vi "Customer-Panel.vi"() -> ()   [LabVIEW 2021]
uses:
  Global-Var-Simulator.vi
panel:
  out "dry_n_shine_ind":bool
  out "rinse_ind":bool
  out "soap_wash_ind":bool
  out "init_wash_ind":bool
  out "none_wash_ind":bool
  out "is_alarm_state_L":bool
  out "is_running_L":bool
  in  "none_wash_opt_btn":bool
  in  "dry_and_shine_opt_btn":bool
  in  "rinse_opt_btn":bool
  in  "soap_wash_opt_btn":bool
  in  "initial_wash_opt_btn":bool
  in  "stop_wash_btn":bool
  in  "start_wash_btn":bool
  out "seconds_ind":dbl
  out "minutes_ind":dbl
  in  "change_collect_btn":bool
  out "is_change_ready_to_collect":bool
  out "change_out_ind":dbl format="%#.2g"
  in  "home_btn":bool
  in  "cash_cancel_btn":bool
  in  "cash_accept_btn":bool
  out "cash_in_ind":dbl format="%#.2g"
  in  "add_cash_5zl_btn":bool
  in  "add_cash_2zl_btn":bool
  in  "add_cash_1zl_btn":bool
  in  "add_chash_50gr_btn":bool
  # "Alarm"
  # "Pozostały czas"
  # "sek"
  # "min"
  # "Tryby mycia"
  # "zł"
  # "Reszta do\nodbioru"
  # "zł"
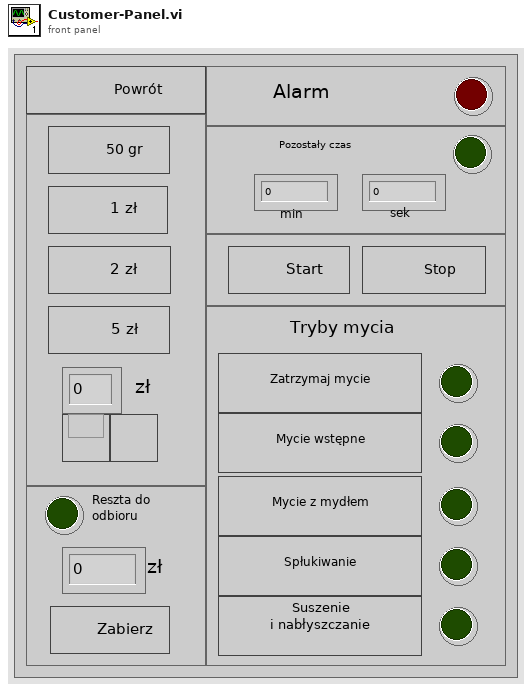
[diagram p1: front panel]
types:
  T1 = enum32{"Invalid", "Standard", "Closed", "Hidden", "Minimized", "Maximized"}
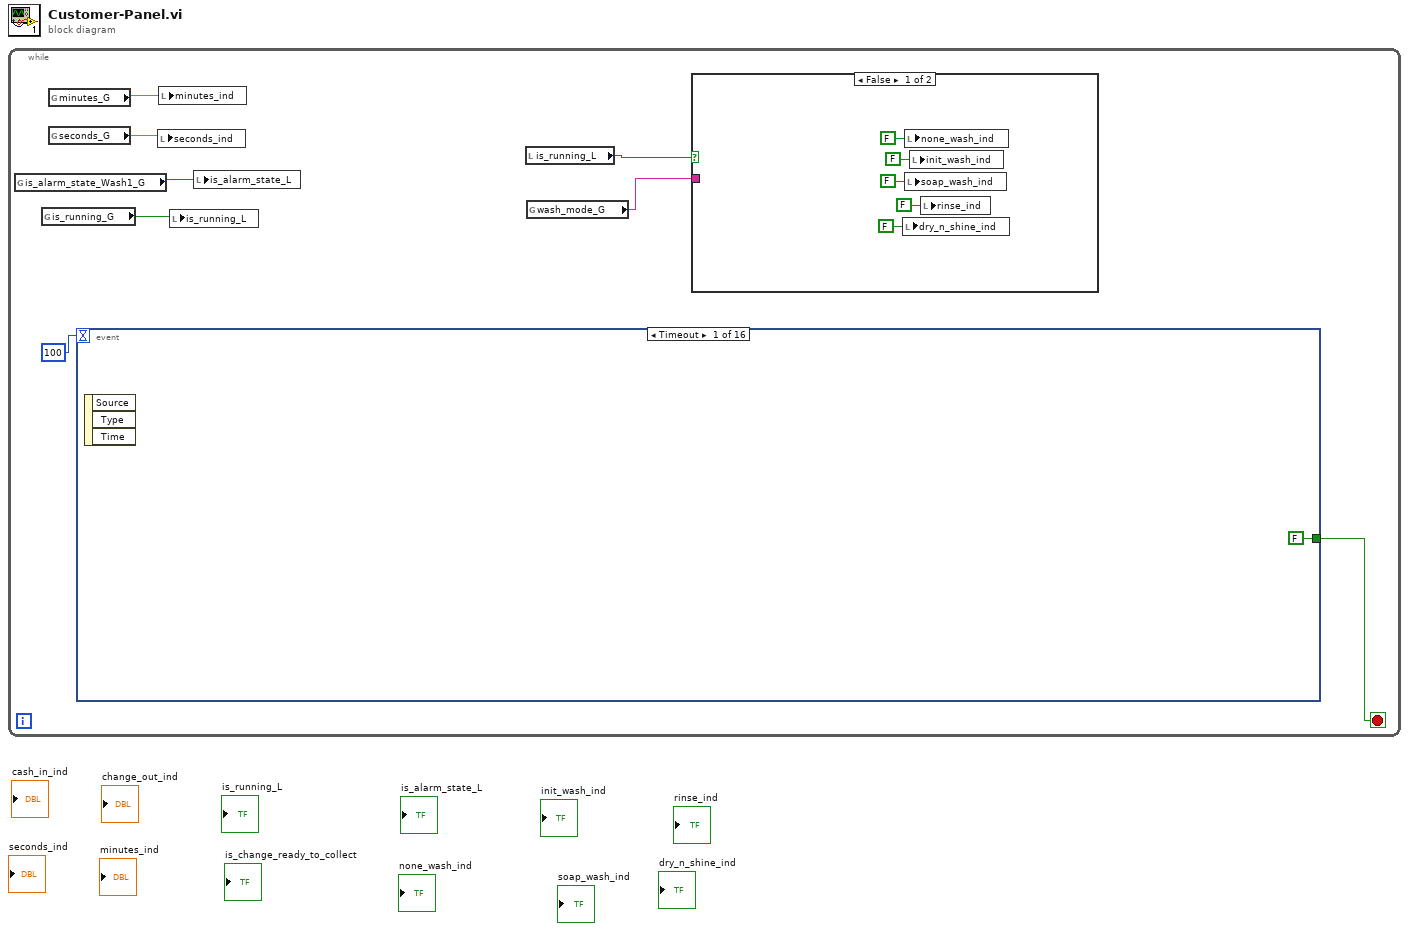
[diagram p0: block diagram]
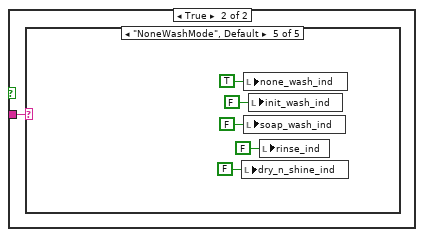
[diagram p2: hidden frame]
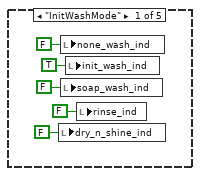
[diagram p3: hidden frame]
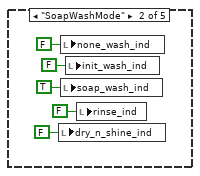
[diagram p4: hidden frame]
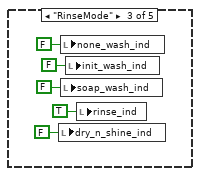
[diagram p5: hidden frame]
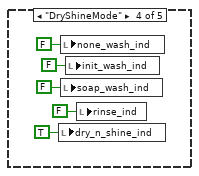
[diagram p6: hidden frame]
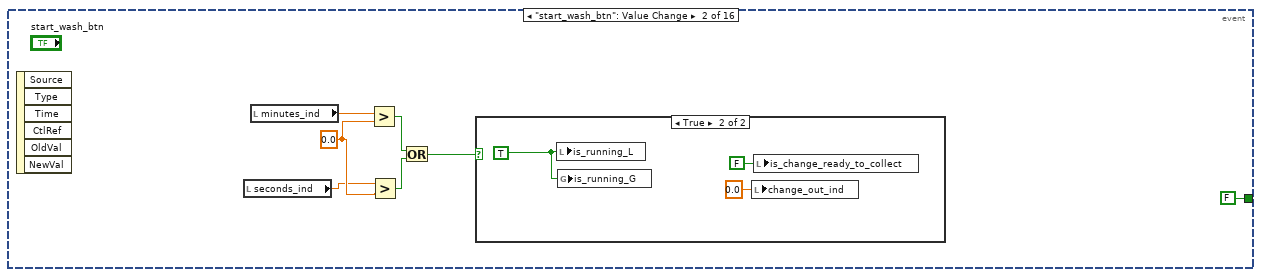
[diagram p7: hidden frame]
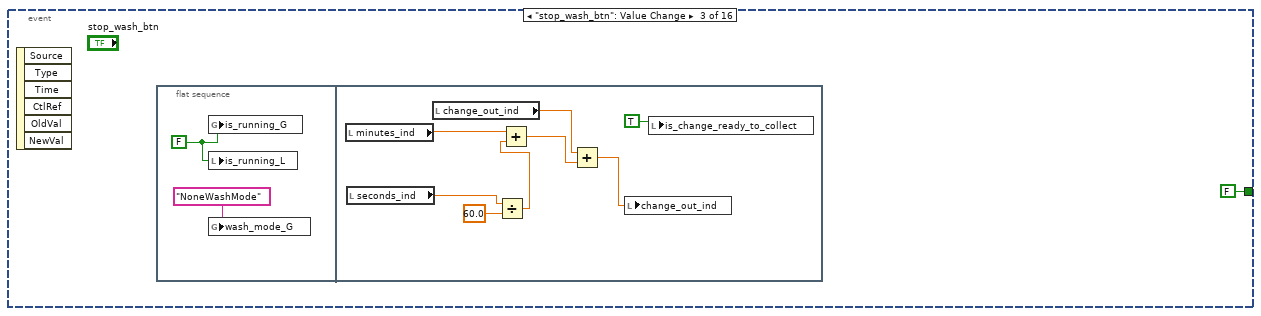
[diagram p9: hidden frame]
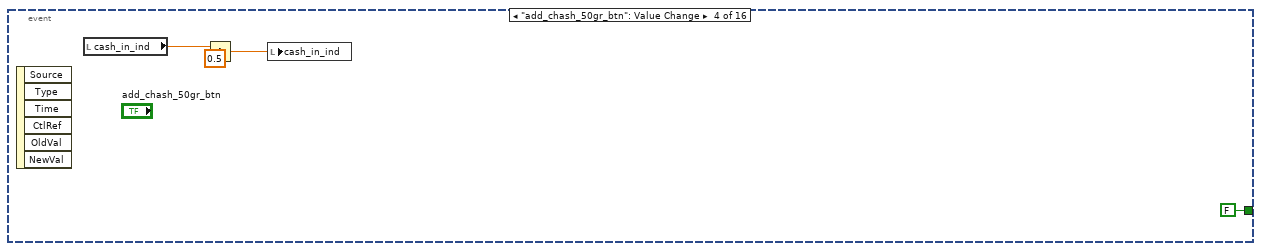
[diagram p10: hidden frame]
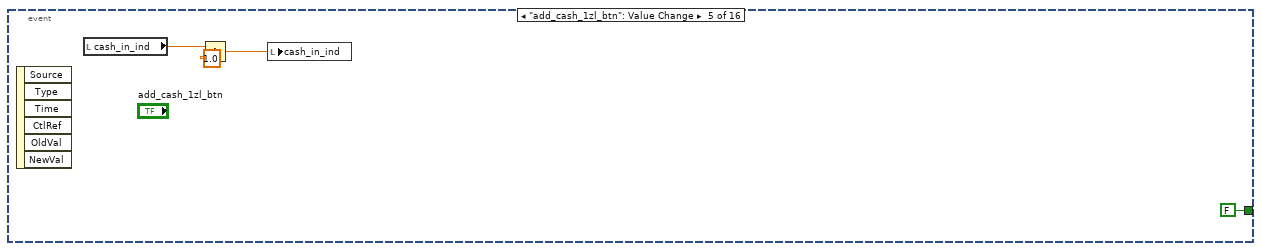
[diagram p11: hidden frame]
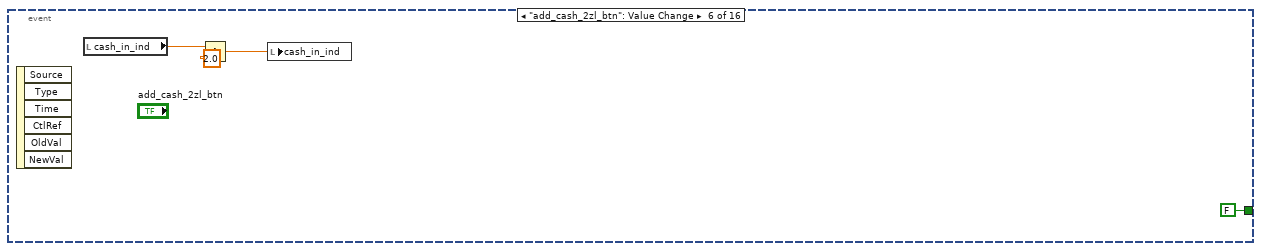
[diagram p12: hidden frame]
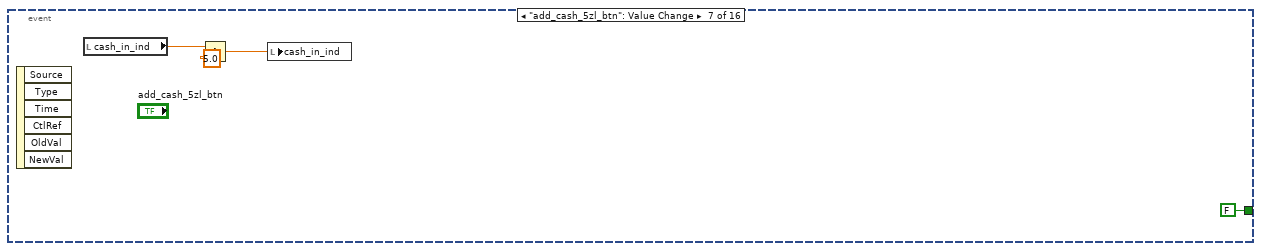
[diagram p13: hidden frame]
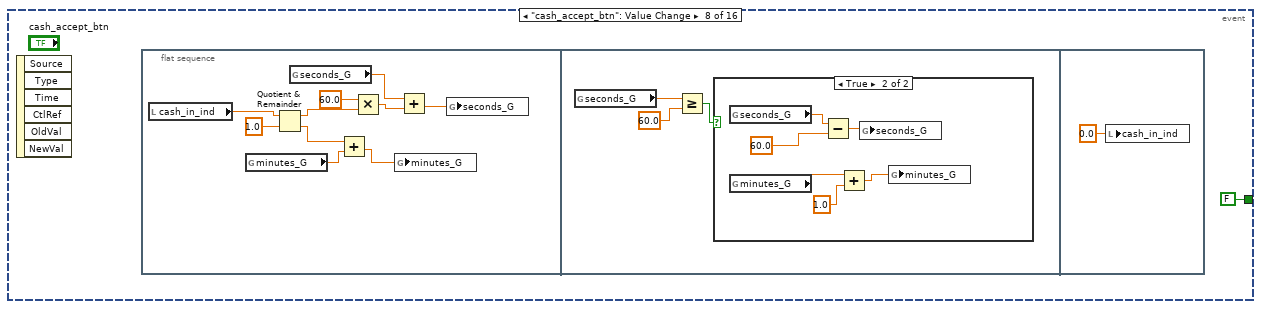
[diagram p14: hidden frame]
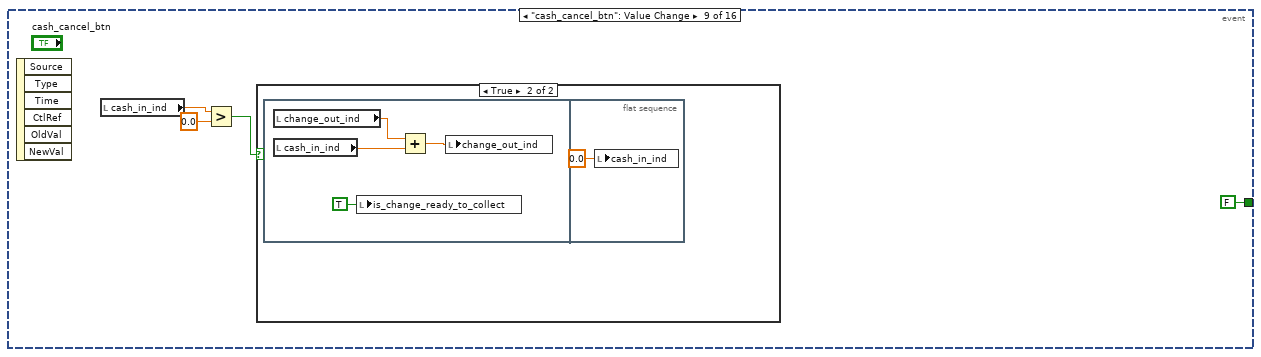
[diagram p16: hidden frame]
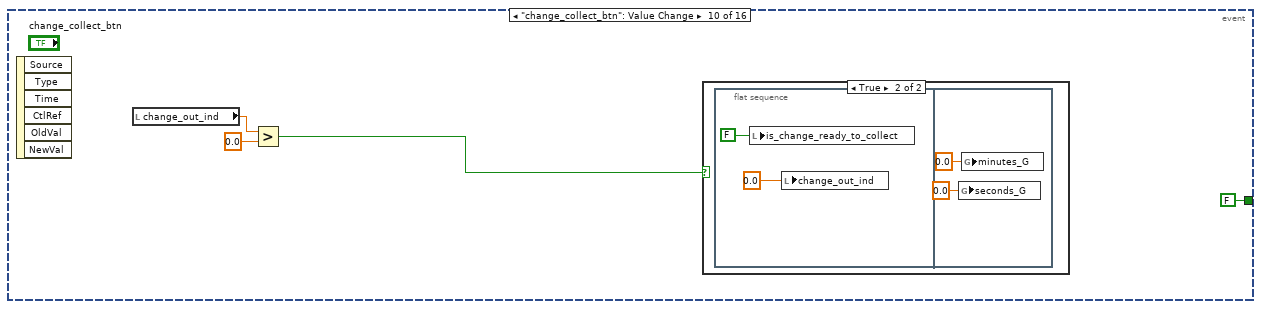
[diagram p18: hidden frame]
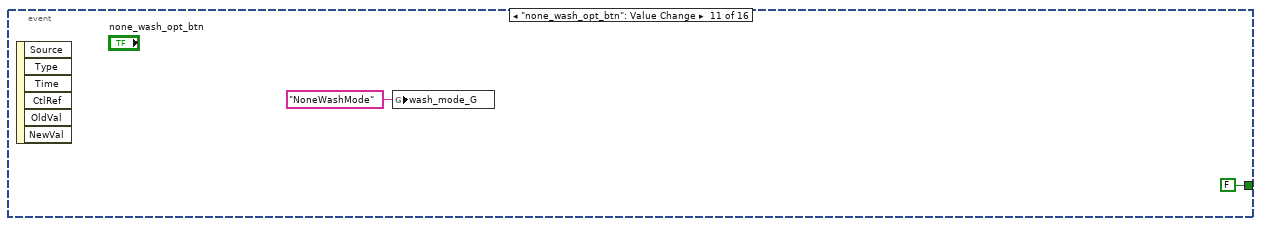
[diagram p20: hidden frame]
diagram:
  n1 = while {
    stop <- w3 stop-if-true
    n2 = global read "Global-Var-Simulator.vi" "is_alarm_state_Wash1_G"() -> (w5:bool)
    n3 = global read "Global-Var-Simulator.vi" "is_running_G"() -> (w4:bool)
    n4 = global read "Global-Var-Simulator.vi" "minutes_G"() -> (w7:dbl)
    n5 = global read "Global-Var-Simulator.vi" "seconds_G"() -> (w6:dbl)
    n6 = event shown="[0] Timeout" {
      selector: _ -> [_ _ _ _ _ _ _ _ _ _ _ _ _ _ _ _]
      dyn-events: _ -> [_ _ _ _ _ _ _ _ _ _ _ _ _ _ _ _]
      timeout: 100 -> [_ _ _ _ _ _ _ _ _ _ _ _ _ _ _ _]
      tunnel: [FALSE FALSE FALSE FALSE FALSE FALSE FALSE FALSE FALSE FALSE FALSE FALSE FALSE FALSE FALSE w126] -> w3
      event Timeout {
        n7 = event-data() -> ()  [unwired: 1 in, 3 out]
      }
      event "start_wash_btn": Value Change {
        w43 = 0.0 ("y")
        n8 = event-data() -> ()  [unwired: 1 in, 6 out]
        n9 = local read "seconds_ind"() -> (w42:dbl)
        n10 = local read "minutes_ind"() -> (w47:dbl)
        n11 = Greater?(x=w47, y=w43) -> (0:w45:bool)
        n12 = Greater?(x=w42, y=w43) -> (0:w46:bool)
        n13 = Or(x=w45, y=w46) -> (x .or. y?=w44:bool)
        n14 = case shown="True" w44 {
          frame False {
          }
          frame True {
            w50 = TRUE ("is_running_L")
            n15 = local write "is_running_L"(w50) -> ()
            n16 = global write "Global-Var-Simulator.vi" "is_running_G"(w50) -> ()
            n17 = local write "change_out_ind"(0.0 ("change_out_ind")) -> ()
            n18 = local write "is_change_ready_to_collect"(FALSE ("is_change_ready_to_collect")) -> ()
          }
        }
      }
      event "stop_wash_btn": Value Change {
        n19 = event-data() -> ()  [unwired: 1 in, 6 out]
        n20 = flat-sequence {
          frame #0 {
            w53 = FALSE ("is_running_G")
            n21 = global write "Global-Var-Simulator.vi" "is_running_G"(w53) -> ()
            n22 = local write "is_running_L"(w53) -> ()
            n23 = global write "Global-Var-Simulator.vi" "wash_mode_G"("NoneWashMode") -> ()
          }
          frame #1 {
            n24 = local read "minutes_ind"() -> (w60:dbl)
            n25 = local read "seconds_ind"() -> (w58:dbl)
            n26 = local read "change_out_ind"() -> (w54:dbl)
            n27 = Divide(x=w58, y=60.0) -> (x/y=w59:dbl)
            n28 = Add(x=w60, y=w59) -> (x+y=w56:dbl)
            n29 = Add(x=w54, y=w56) -> (x+y=w55:dbl)
            n30 = local write "change_out_ind"(w55) -> ()
            n31 = local write "is_change_ready_to_collect"(TRUE ("is_change_ready_to_collect")) -> ()
          }
        }
      }
      event "add_chash_50gr_btn": Value Change {
        n32 = event-data() -> ()  [unwired: 1 in, 6 out]
        n33 = local read "cash_in_ind"() -> (w63:dbl)
        n34 = Add(x=w63, y=0.5) -> (x+y=w64:dbl)
        n35 = local write "cash_in_ind"(w64) -> ()
      }
      event "add_cash_1zl_btn": Value Change {
        n36 = event-data() -> ()  [unwired: 1 in, 6 out]
        n37 = local read "cash_in_ind"() -> (w67:dbl)
        n38 = Add(x=w67, y=1.0) -> (x+y=w68:dbl)
        n39 = local write "cash_in_ind"(w68) -> ()
      }
      event "add_cash_2zl_btn": Value Change {
        n40 = event-data() -> ()  [unwired: 1 in, 6 out]
        n41 = local read "cash_in_ind"() -> (w71:dbl)
        n42 = Add(x=w71, y=2.0) -> (x+y=w72:dbl)
        n43 = local write "cash_in_ind"(w72) -> ()
      }
      event "add_cash_5zl_btn": Value Change {
        n44 = event-data() -> ()  [unwired: 1 in, 6 out]
        n45 = local read "cash_in_ind"() -> (w75:dbl)
        n46 = Add(x=w75, y=5.0) -> (x+y=w76:dbl)
        n47 = local write "cash_in_ind"(w76) -> ()
      }
      event "cash_accept_btn": Value Change {
        n48 = event-data() -> ()  [unwired: 1 in, 6 out]
        n49 = flat-sequence {
          frame #0 {
            n50 = local read "cash_in_ind"() -> (w88:dbl)
            n51 = global read "Global-Var-Simulator.vi" "minutes_G"() -> (w82:dbl)
            n52 = Quotient & Remainder(x=w88, y=1.0) -> (x-y*floor(x/y)=w85:dbl, floor(x/y)=w86:dbl)
            n53 = global read "Global-Var-Simulator.vi" "seconds_G"() -> (w80:dbl)
            n54 = Add(x=w86, y=w82) -> (x+y=w81:dbl)
            n55 = Multiply(x=60.0, y=w85) -> (x*y=w83:dbl)
            n56 = global write "Global-Var-Simulator.vi" "minutes_G"(w81) -> ()
            n57 = Add(x=w80, y=w83) -> (x+y=w79:dbl)
            n58 = global write "Global-Var-Simulator.vi" "seconds_G"(w79) -> ()
          }
          frame #1 {
            n59 = global read "Global-Var-Simulator.vi" "seconds_G"() -> (w91:dbl)
            n60 = Greater Or Equal?(x=w91, y=60.0) -> (x >= y?=w89:bool)
            n61 = case shown="True" w89 {
              frame False {
              }
              frame True {
                n62 = global read "Global-Var-Simulator.vi" "seconds_G"() -> (w97:dbl)
                n63 = global read "Global-Var-Simulator.vi" "minutes_G"() -> (w93:dbl)
                n64 = Subtract(x=w97, y=60.0) -> (x-y=w95:dbl)
                n65 = Add(x=w93, y=1.0) -> (x+y=w94:dbl)
                n66 = global write "Global-Var-Simulator.vi" "seconds_G"(w95) -> ()
                n67 = global write "Global-Var-Simulator.vi" "minutes_G"(w94) -> ()
              }
            }
          }
          frame #2 {
            n68 = local write "cash_in_ind"(0.0 ("cash_in_ind")) -> ()
          }
        }
      }
      event "cash_cancel_btn": Value Change {
        n69 = event-data() -> ()  [unwired: 1 in, 6 out]
        n70 = local read "cash_in_ind"() -> (w102:dbl)
        n71 = Greater?(x=w102, y=0.0) -> (0:w100:bool)
        n72 = case shown="True" w100 {
          frame False {
          }
          frame True {
            n73 = flat-sequence {
              frame #0 {
                n74 = local read "change_out_ind"() -> (w103:dbl)
                n75 = local read "cash_in_ind"() -> (w104:dbl)
                n76 = local write "is_change_ready_to_collect"(TRUE ("is_change_ready_to_collect")) -> ()
                n77 = Add(x=w103, y=w104) -> (x+y=w105:dbl)
                n78 = local write "change_out_ind"(w105) -> ()
              }
              frame #1 {
                n79 = local write "cash_in_ind"(0.0 ("cash_in_ind")) -> ()
              }
            }
          }
        }
      }
      event "change_collect_btn": Value Change {
        n80 = event-data() -> ()  [unwired: 1 in, 6 out]
        n81 = local read "change_out_ind"() -> (w111:dbl)
        n82 = Greater?(x=w111, y=0.0) -> (0:w109:bool)
        n83 = case shown="True" w109 {
          frame False {
          }
          frame True {
            n84 = flat-sequence {
              frame #0 {
                n85 = local write "is_change_ready_to_collect"(FALSE ("is_change_ready_to_collect")) -> ()
                n86 = local write "change_out_ind"(0.0 ("change_out_ind")) -> ()
              }
              frame #1 {
                n87 = global write "Global-Var-Simulator.vi" "seconds_G"(0.0 ("seconds_G")) -> ()
                n88 = global write "Global-Var-Simulator.vi" "minutes_G"(0.0 ("minutes_G")) -> ()
              }
            }
          }
        }
      }
      event "none_wash_opt_btn": Value Change {
        n89 = event-data() -> ()  [unwired: 1 in, 6 out]
        n90 = global write "Global-Var-Simulator.vi" "wash_mode_G"("NoneWashMode" ("wash_mode_G")) -> ()
      }
      event "initial_wash_opt_btn": Value Change {
        n91 = event-data() -> ()  [unwired: 1 in, 6 out]
        n92 = global write "Global-Var-Simulator.vi" "wash_mode_G"("InitWashMode" ("wash_mode_G")) -> ()
      }
      event "soap_wash_opt_btn": Value Change {
        n93 = event-data() -> ()  [unwired: 1 in, 6 out]
        n94 = global write "Global-Var-Simulator.vi" "wash_mode_G"("SoapWashMode" ("wash_mode_G")) -> ()
      }
      event "rinse_opt_btn": Value Change {
        n95 = event-data() -> ()  [unwired: 1 in, 6 out]
        n96 = global write "Global-Var-Simulator.vi" "wash_mode_G"("RinseMode" ("wash_mode_G")) -> ()
      }
      event "dry_and_shine_opt_btn": Value Change {
        n97 = event-data() -> ()  [unwired: 1 in, 6 out]
        n98 = global write "Global-Var-Simulator.vi" "wash_mode_G"("DryShineMode" ("wash_mode_G")) -> ()
      }
      event "home_btn": Value Change {
        n99 = event-data() -> ()  [unwired: 1 in, 6 out]
        n100 = flat-sequence {
          tunnel: [TRUE] -> w126
          frame #0 {
            n101 = call "OpenPanel(SubVI).vi"("String"="Login-Panel.vi", "State"=T1."Maximized", "Wait Until Done"=FALSE, "Auto Dispose Reference"=FALSE) -> ()  [unwired: 8 in]
          }
          frame #1 {
            n102 = call "ClosePanel(SubVI).vi"("String"="Customer-Panel.vi") -> ()  [unwired: 11 in]
          }
          frame #2 {
          }
        }
      }
    }
    n103 = local write "seconds_ind"(w6) -> ()
    n104 = local write "minutes_ind"(w7) -> ()
    n105 = local write "is_running_L"(w4) -> ()
    n106 = local write "is_alarm_state_L"(w5) -> ()
    n107 = local read "is_running_L"() -> (w2:bool)
    n108 = global read "Global-Var-Simulator.vi" "wash_mode_G"() -> (w1:string)
    n109 = case shown="False" w2 {
      tunnel: w1 -> [_ w14]
      frame False {
        n110 = local write "dry_n_shine_ind"(FALSE ("dry_n_shine_ind")) -> ()
        n111 = local write "none_wash_ind"(FALSE ("none_wash_ind")) -> ()
        n112 = local write "soap_wash_ind"(FALSE ("soap_wash_ind")) -> ()
        n113 = local write "init_wash_ind"(FALSE ("init_wash_ind")) -> ()
        n114 = local write "rinse_ind"(FALSE ("rinse_ind")) -> ()
      }
      frame True {
        n115 = case shown="\"NoneWashMode\", Default" w14 {
          frame "InitWashMode" {
            n116 = local write "dry_n_shine_ind"(FALSE ("dry_n_shine_ind")) -> ()
            n117 = local write "none_wash_ind"(FALSE ("none_wash_ind")) -> ()
            n118 = local write "soap_wash_ind"(FALSE ("soap_wash_ind")) -> ()
            n119 = local write "init_wash_ind"(TRUE ("init_wash_ind")) -> ()
            n120 = local write "rinse_ind"(FALSE ("rinse_ind")) -> ()
          }
          frame "SoapWashMode" {
            n121 = local write "dry_n_shine_ind"(FALSE ("dry_n_shine_ind")) -> ()
            n122 = local write "none_wash_ind"(FALSE ("none_wash_ind")) -> ()
            n123 = local write "soap_wash_ind"(TRUE ("soap_wash_ind")) -> ()
            n124 = local write "init_wash_ind"(FALSE ("init_wash_ind")) -> ()
            n125 = local write "rinse_ind"(FALSE ("rinse_ind")) -> ()
          }
          frame "RinseMode" {
            n126 = local write "dry_n_shine_ind"(FALSE ("dry_n_shine_ind")) -> ()
            n127 = local write "none_wash_ind"(FALSE ("none_wash_ind")) -> ()
            n128 = local write "soap_wash_ind"(FALSE ("soap_wash_ind")) -> ()
            n129 = local write "init_wash_ind"(FALSE ("init_wash_ind")) -> ()
            n130 = local write "rinse_ind"(TRUE ("rinse_ind")) -> ()
          }
          frame "DryShineMode" {
            n131 = local write "dry_n_shine_ind"(TRUE ("dry_n_shine_ind")) -> ()
            n132 = local write "none_wash_ind"(FALSE ("none_wash_ind")) -> ()
            n133 = local write "soap_wash_ind"(FALSE ("soap_wash_ind")) -> ()
            n134 = local write "init_wash_ind"(FALSE ("init_wash_ind")) -> ()
            n135 = local write "rinse_ind"(FALSE ("rinse_ind")) -> ()
          }
          frame "NoneWashMode", Default {
            n136 = local write "dry_n_shine_ind"(FALSE ("dry_n_shine_ind")) -> ()
            n137 = local write "none_wash_ind"(TRUE ("none_wash_ind")) -> ()
            n138 = local write "soap_wash_ind"(FALSE ("soap_wash_ind")) -> ()
            n139 = local write "init_wash_ind"(FALSE ("init_wash_ind")) -> ()
            n140 = local write "rinse_ind"(FALSE ("rinse_ind")) -> ()
          }
        }
      }
    }
  }
